vi "Create New.vi"(0 "Display State In":T1={"Item_Refnums_Array"=[], "Root Command"={"Operation"=enum."Add Item", "Data"=variant}}, 9 "Container State":T6, 11 "error in (no error)":errorcluster) -> (4 "Display State Out":T1={"Item_Refnums_Array"=[], "Root Command"={"Operation"=enum."Add Item", "Data"=variant}}, 15 "error out":errorcluster)   [LabVIEW 2011, in "Root_XControl.xctl"]
uses:
  Root_XControl.xctl
  <vilib>/_xctls/Container State.ctl
  State 1.ctl
  Controls/References/Item_Refnums.ctl
  Controls/References/Item_Command_Refnum.ctl
  Controls/Item_Command_Enum.ctl
  Controls/Root_Command.ctl
  Controls/Root_Command_Enum.ctl
  <vilib>/_xctls/XControlSupport.lvlib
types:
  T1 = typedef "Root_XControl.xctl/State 1.ctl" = cluster{"Item_Refnums_Array":T2[], "Root Command":T4}
  T2 = typedef "Item_Refnums.ctl" = cluster{"VI Refnum":refnum<vi>, "Item_Command_Refnum":T3, "Slide Refnum":refnum<vi>}
  T3 = typedef "Item_Command_Refnum.ctl" = refnum<vi>
  T4 = typedef "Root_Command.ctl" = cluster{"Operation":T5, "Data":variant}
  T5 = typedef "Root_Command_Enum.ctl" = enum16{"Idle", "Add Item", "Delete Item", "Delete All"}
  T6 = typedef "XControlSupport.lvlib/Container State.ctl" = cluster{"Indicator?":bool, "Run Mode?":bool, " Refnum":refnum<vi>}
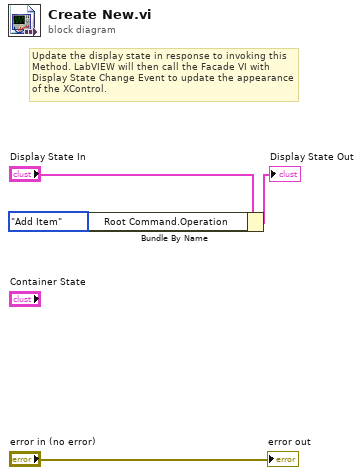
[diagram p0: block diagram]
diagram:
  # "Update the display state in response to invoking this Method. LabVIEW will then call the Facade VI with Display State Change Event to update the appearance of the XControl."
  n1 = Bundle By Name(cluster="Display State In", "Root Command.Operation"=Root_Command_Enum."Add Item" ("Enum")) -> (→"Display State Out":T1)
  "error out" <- "error in (no error)"
